vi "Save Epics Configuration.vi"(8 "error in (no error)":errorcluster, 11 "Master Configuration in":T1) -> (0 "error out":errorcluster, 3 "Master Configuration out":T1)   [LabVIEW 2014]
uses:
  controls/Master Configuration.ctl
  controls/EPICS Configuration.ctl
  <vilib>/Utility/config.llb/NI_LVConfig.lvlib
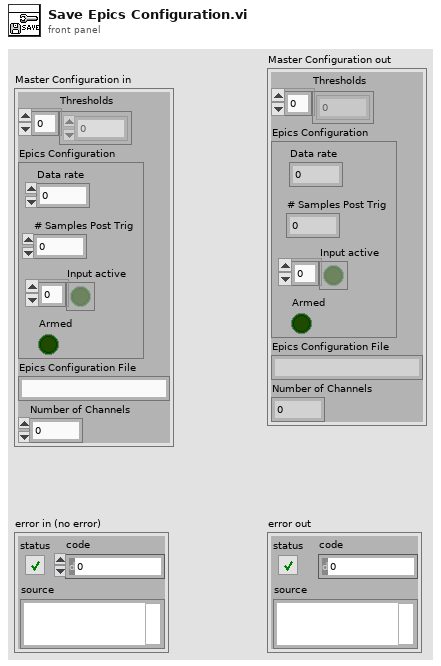
[diagram p1: front panel]
types:
  T1 = typedef "Master Configuration.ctl" = cluster{"Thresholds":dbl[], "Epics Configuration":T2, "Epics Configuration File":string, "Number of Channels":dbl}
  T2 = typedef "EPICS Configuration.ctl" = cluster{"Data rate":u32, "Input active":bool[], "# Samples Post Trig":u32, "Armed":bool}
  T3 = typedef "NI_LVConfig.lvlib/Config Data RefNum.ctl" = refnum<k1>
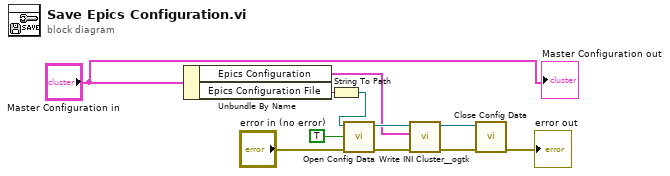
[diagram p0: block diagram]
diagram:
  n1 = Unbundle By Name("Master Configuration in") -> ("Epics Configuration"=w6:T2, "Epics Configuration File"=w2:string)
  n2 = String To Path(string=w2) -> (path=w3:path)
  n3 = call <vilib>:"Open Config Data.vi"("error in (no error)"="error in (no error)", "create file if necessary (T)"=TRUE, "configuration file path"=w3) -> ("error out"=w1:errorcluster, "refnum"=w7:T3)  [unwired: 6 in, 1 out]
  n4 = call <userlib>:"Write INI Cluster__ogtk.vi"("error in (no error)"=w1, "INI Fomatted Cluster"=w6, "refnum"=w7) -> ("error out"=w5:errorcluster, "dup refnum"=w8:T3)  [unwired: 7 in]
  n5 = call <vilib>:"Close Config Data.vi"("error in (no error)"=w5, "refnum"=w8) -> ("error out"=→"error out":errorcluster)  [unwired: 8 in, 1 out]
  "Master Configuration out" <- "Master Configuration in"
